vi "Load Debug Snapshot.vi"(6 "IPath Getter in":refnum<class "IPath Getter.lvclass">, 8 "error in":errorcluster, 10 "Debug Elements Options":T1={"Breakpoints"=TRUE, "Probes"=TRUE}, 11 "VI Reference in":refnum<vi>) -> (0 "error out":errorcluster, 2 "VI Debug Elements":T2, 3 "VI Reference out":refnum<vi>)   [LabVIEW 2020]
doc: "Load <b>Debug Snapshot</b> of the active VI from Cache File."
uses:
  Type Definitions/Debug Snapshot--cluster.ctl
  Type Definitions/Breakpoint--cluster.ctl
  <vilib>/Utility/miscctls.llb/LVBreakpointStatusEnum.ctl
  Type Definitions/Class Name--enum.ctl
  Type Definitions/Snapshot Handling Options--cluster.ctl
  IPath Getter/IPath Getter.lvclass
  Type Definitions/Debug Snapshot Array--cluster.ctl
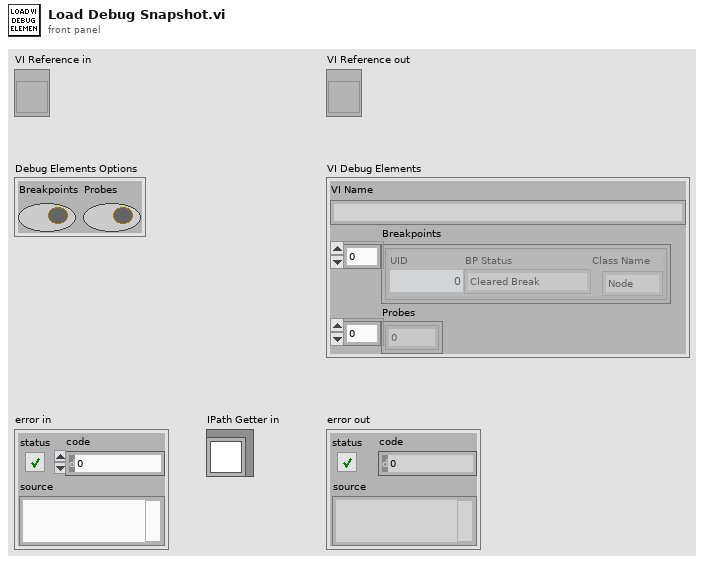
[diagram p1: front panel]
types:
  T1 = typedef "Snapshot Handling Options--cluster.ctl" = cluster{"Breakpoints":bool, "Probes":bool}
  T2 = typedef "Debug Snapshot--cluster.ctl" = cluster{"VI Name":string, "Breakpoints":T3[], "Probes":i32[]}
  T3 = typedef "Breakpoint--cluster.ctl" = cluster{"UID":i32, "BP Status":T4, "Class Name":T5}
  T4 = typedef "LVBreakpointStatusEnum.ctl" = enum8{"Cleared Break", "Enabled Break", "Disabled Break"}
  T5 = typedef "Class Name--enum.ctl" = enum16{"Node", "Wire"}
  T6 = typedef "Debug Snapshot Array--cluster.ctl" = cluster{"Debug Snapshots":T2[]}
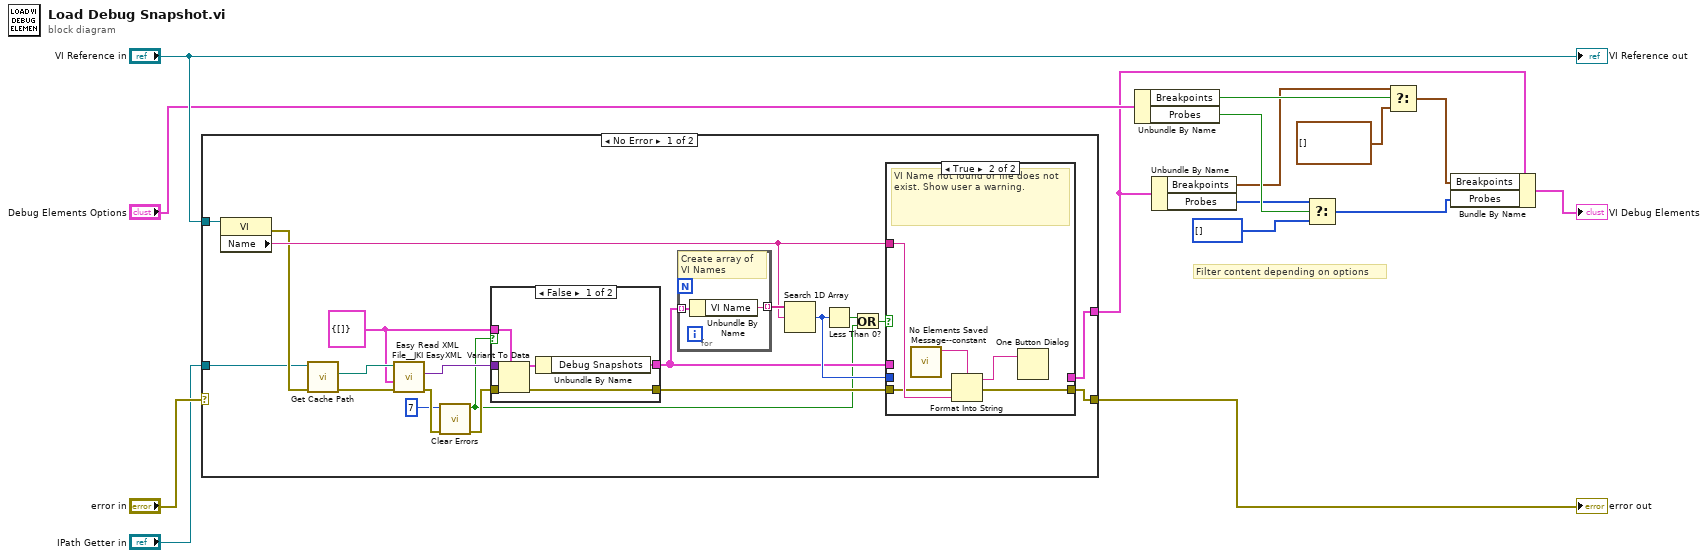
[diagram p0: block diagram]
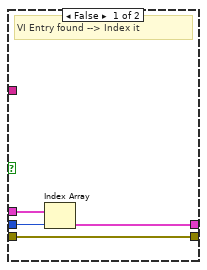
[diagram p3: hidden frame]
diagram:
  # "Filter content depending on options"
  n1 = case shown="No Error" "error in" {
    selector: "error in" -> [_ w54]
    tunnel: [w29 w54] -> w14
    tunnel: "VI Reference in" -> [w35 _]
    tunnel: [w28 _] -> w5
    tunnel: "IPath Getter in" -> [w24 _]
    frame No Error {
      w23 = T6 {"Debug Snapshots"=[]} ("Debug Snapshots_")
      n2 = property class="VI"(reference=w35) -> (error out=w27:errorcluster, "Name"=w31:string)  [unwired: 1 in, 1 out]
      n3 = call-dynamic "Get Cache Path.vi"("error in (no error)"=w27, "IPath Getter in"=w24) -> ("error out"=w26:errorcluster, "Path"=w25:path)  [unwired: 8 in]
      n4 = call <vilib>:"Easy Read XML File__JKI EasyXML.vi"("error in (no error)"=w26, "LabVIEW Data (Type)"=w23, "XML File Path"=w25) -> ("error out"=w21:errorcluster, "LabVIEW Data"=w34:variant)  [unwired: 6 in, 1 out]
      n5 = call <vilib>:"Clear Errors.vi"("error in (no error)"=w21, "specific error code to clear (0: all)"=7) -> ("error out"=w20:errorcluster, "specific error cleared?"=w16:bool)  [unwired: 4 in]
      n6 = case shown="False" w16 {
        tunnel: w34 -> [w41 _]
        tunnel: [w40 w42] -> w30
        tunnel: w23 -> [w39 _]
        tunnel: [w37 _] -> w22
        tunnel: w20 -> [w36 w42]
        frame False {
          n7 = Variant To Data(error in=w36, type=w39, Variant=w41) -> (data=w38:T6, error out=w40:errorcluster)
          n8 = Unbundle By Name(w38) -> ("Debug Snapshots"=w37:T2[])
        }
        frame True {
        }
      }
      n9 = for {
        tunnel: w22 -> [w53] mode=indexing
        tunnel: [w52] -> w33 mode=indexing
        # "Create array of\nVI Names"
        n10 = Unbundle By Name(w53) -> ("VI Name"=w52:string)
      }
      n11 = Search 1D Array(1D array=w33, element=w31) -> (index of element=w32:i32)  [unwired: 1 in]
      n12 = Less Than 0?(x=w32) -> (x < 0?=w18:bool)
      n13 = Or(x=w18, y=w16) -> (x .or. y?=w17:bool)
      n14 = case shown="True" w17 {
        tunnel: w22 -> [w46 _]
        tunnel: w32 -> [w45 _]
        tunnel: w31 -> [_ w50]
        tunnel: w30 -> [w44 w48]
        tunnel: [w44 w47] -> w29
        tunnel: [w43 _] -> w28
        frame False {
          # "VI Entry found --> Index it"
          n15 = Index Array(array=w46, index=w45) -> (element=w43:T2)
        }
        frame True {
          # "VI Name not found or file does not exist. Show user a warning."
          n16 = call "No Elements Saved Message--constant.vi"() -> ("message"=w51:string)  [unwired: 11 in]
          n17 = Format Into String(format string=w51, error in=w48, w50) -> (resulting string=w49:string, error out=w47:errorcluster)  [unwired: 1 in]
          n18 = One Button Dialog(message=w49) -> ()  [unwired: 1 in, 1 out]
        }
      }
    }
    frame Error {
      # "Pass error without further action"
    }
  }
  "error out" <- w14
  n19 = Unbundle By Name("Debug Elements Options") -> ("Breakpoints"=w11:bool, "Probes"=w10:bool)
  n20 = Unbundle By Name(w5) -> ("Breakpoints"=w9:T3[], "Probes"=w8:i32[])
  n21 = Select(t=w8, s=w10, f=i32[] []) -> (s? t:f=w3:i32[])
  n22 = Select(t=w9, s=w11, f=T3[] []) -> (s? t:f=w4:T3[])
  n23 = Bundle By Name(cluster=w5, "Breakpoints"=w4, "Probes"=w3) -> (→"VI Debug Elements":T2)
  "VI Reference out" <- "VI Reference in"
